vi "Request Address and Name.vi"(11 "Nodes":T1[](array[typedef]) {"Name" format="%.0x"}) -> (2 "Cancel out":bool, 3 "J1939 Monitor Settings":T1 {"Name" format="%.0x"})   [LabVIEW 2023, in "J1939 Addon System Explorer.lvlib"]
uses:
  J1939 Addon System Explorer.lvlib
  Addon Shared/Types/Monitor Settings.ctl
  Addon Shared/J1939 Addon Shared.lvlib
panel:
  in  "Name":u64=1 format="%.0x"
  in  "Address":u8 format="%.0x"
  in  "Cancel":bool
  in  "Select":bool
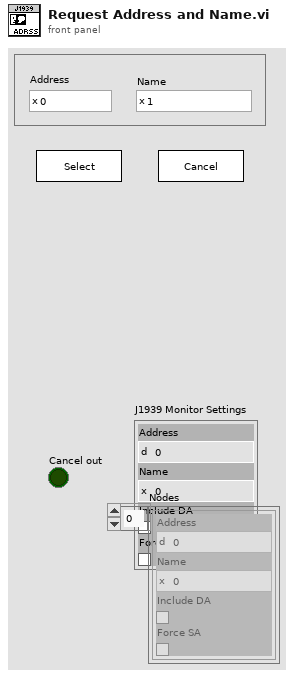
[diagram p1: front panel]
types:
  T1 = typedef "J1939 Addon Shared.lvlib/Monitor Settings.ctl" = cluster{"Address":u8, "Name":u64, "Include DA":bool, "Force SA":bool}
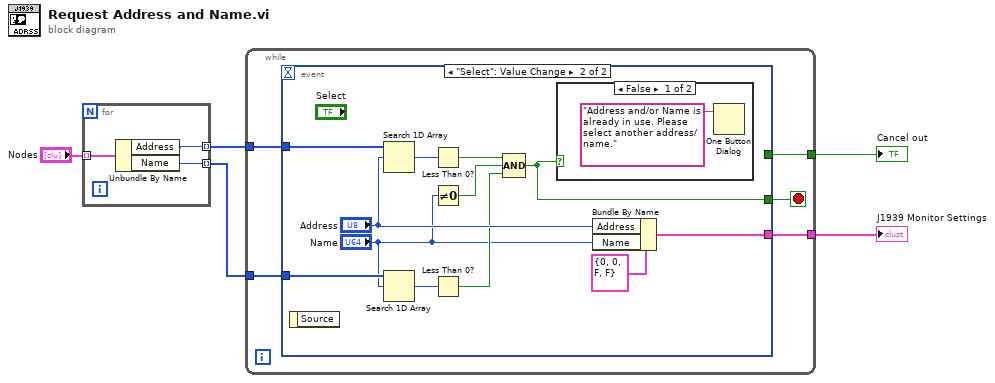
[diagram p0: block diagram]
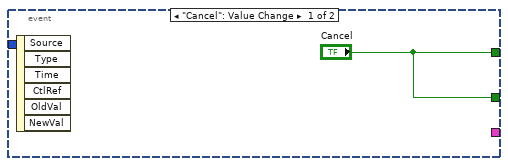
[diagram p2: hidden frame]
diagram:
  n1 = for {
    tunnel: "Nodes" -> [w8] mode=indexing
    tunnel: [w7] -> w2 mode=indexing
    tunnel: [w6] -> w1 mode=indexing
    n2 = Unbundle By Name(w8) -> ("Address"=w7:u8, "Name"=w6:u64)
  }
  n3 = while {
    tunnel: [w13] -> w5
    tunnel: [w12] -> w4
    tunnel: w2 -> [w10]
    tunnel: w1 -> [w9]
    stop <- w11 stop-if-true
    n4 = event shown="[1] \"Select\": Value Change" {
      selector: _ -> [_ _]
      dyn-events: _ -> [_ _]
      timeout: _ -> [_ _]
      tunnel: [_ w25] -> w13
      tunnel: ["Cancel" _] -> w12
      tunnel: ["Cancel" w17] -> w11
      tunnel: w10 -> [_ w24]
      tunnel: w9 -> [_ w21]
      event "Cancel": Value Change {
        n5 = event-data() -> ()  [unwired: 1 in, 6 out]
      }
      event "Select": Value Change {
        n6 = event-data() -> ()  [unwired: 1 in, 1 out]
        n7 = Search 1D Array(1D array=w24, element="Address") -> (index of element=w22:i32)  [unwired: 1 in]
        n8 = Search 1D Array(1D array=w21, element="Name") -> (index of element=w20:i32)  [unwired: 1 in]
        n9 = Less Than 0?(x=w22) -> (x < 0?=w18:bool)
        n10 = Not Equal To 0?(x="Name") -> (x != 0?=w15:bool)
        n11 = Less Than 0?(x=w20) -> (x < 0?=w19:bool)
        n12 = Compound Arithmetic op=AND(w18, w15, w19) -> (w17:bool)
        n13 = case shown="False" w17 {
          frame False {
            n14 = One Button Dialog(message="Address and/or Name is already in use. Please select another address/name.") -> ()  [unwired: 1 in, 1 out]
          }
          frame True {
          }
        }
        n15 = Bundle By Name(cluster=T1 {"Address"=0, "Name"=0, "Include DA"=FALSE, "Force SA"=FALSE} ("J1939 Monitor Settings"), "Address"="Address", "Name"="Name") -> (w25:T1)
      }
    }
  }
  "J1939 Monitor Settings" <- w5
  "Cancel out" <- w4
